vi "FlatToRichrfcontrol_USBRequest.vi"(5 "OutputClusterType":T1, 11 "InputCluster":T2) -> (3 "OutputCluster":T1)   [LabVIEW 2024, in "FlexSDR_gRPC_client.lvlib"]
uses:
  rfcontrol_USBRequest_Flat.ctl
  rfcontrol_USBRequest.ctl
  FlexSDR_gRPC_client.lvlib
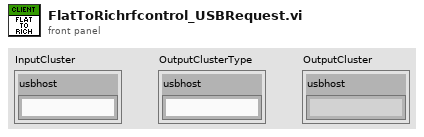
[diagram p1: front panel]
types:
  T1 = typedef "FlexSDR_gRPC_client.lvlib/rfcontrol_USBRequest.ctl" = cluster{"usbhost":string}
  T2 = typedef "FlexSDR_gRPC_client.lvlib/rfcontrol_USBRequest_Flat.ctl" = cluster{"usbhost":string}
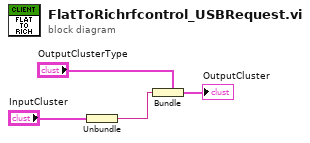
[diagram p0: block diagram]
diagram:
  n1 = Unbundle "Unbundle"("InputCluster") -> ("usbhost"=w1:string)
  n2 = Bundle "Bundle"(cluster="OutputClusterType", "usbhost"=w1) -> (→"OutputCluster":T1)
